vi "Destroy.vi"(8 "error in (no error)":errorcluster, 11 "Gantry Status in":refnum<class "Gantry Status.lvclass">) -> (0 "error out":errorcluster)   [LabVIEW 2017, in "Gantry Status.lvclass"]
uses:
  Gantry Status.lvclass
  Gantry Status.lvclass/Gantry Status.ctl
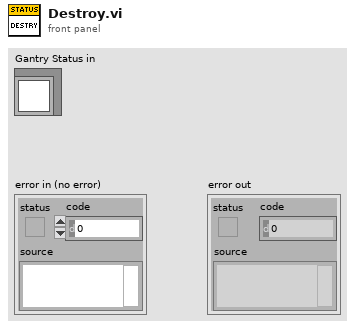
[diagram p1: front panel]
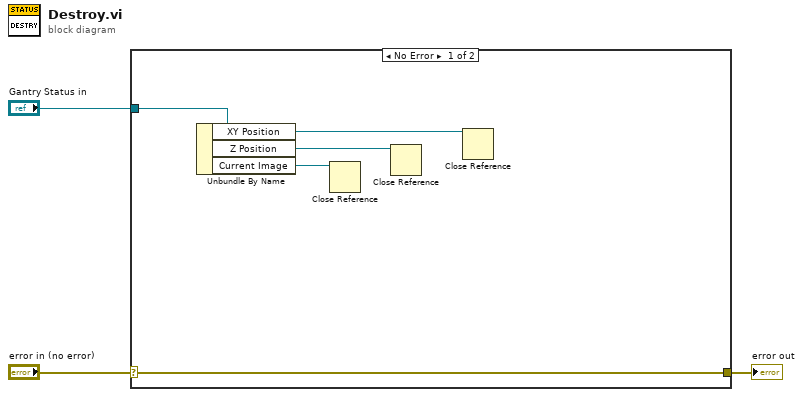
[diagram p0: block diagram]
diagram:
  n1 = case shown="No Error" "error in (no error)" {
    selector: "error in (no error)" -> [w8 w9]
    tunnel: [w8 w9] -> w2
    tunnel: "Gantry Status in" -> [w7 _]
    frame No Error {
      n2 = Unbundle By Name(w7) -> ("XY Position"=w4:refnum<vi>, "Z Position"=w5:refnum<vi>, "Current Image"=w6:refnum<vi>)
      n3 = Close Reference(reference=w6) -> ()  [unwired: 1 in, 1 out]
      n4 = Close Reference(reference=w5) -> ()  [unwired: 1 in, 1 out]
      n5 = Close Reference(reference=w4) -> ()  [unwired: 1 in, 1 out]
    }
    frame Error {
    }
  }
  "error out" <- w2
